vi "Sub05_MatlabFileBuilder.vi"(5 "Select line style":string(combo), 6 "Ball touch color":u32(colorbox), 7 "appended array":T2(array[cluster]), 8 "error in (no error)":errorcluster, 9 "Band touch color":u32(colorbox), 10 "CommandInfo":T1, 11 "Select sequence":string) -> (0 "error out":errorcluster, 3 "Script":string)   [LabVIEW 2019]
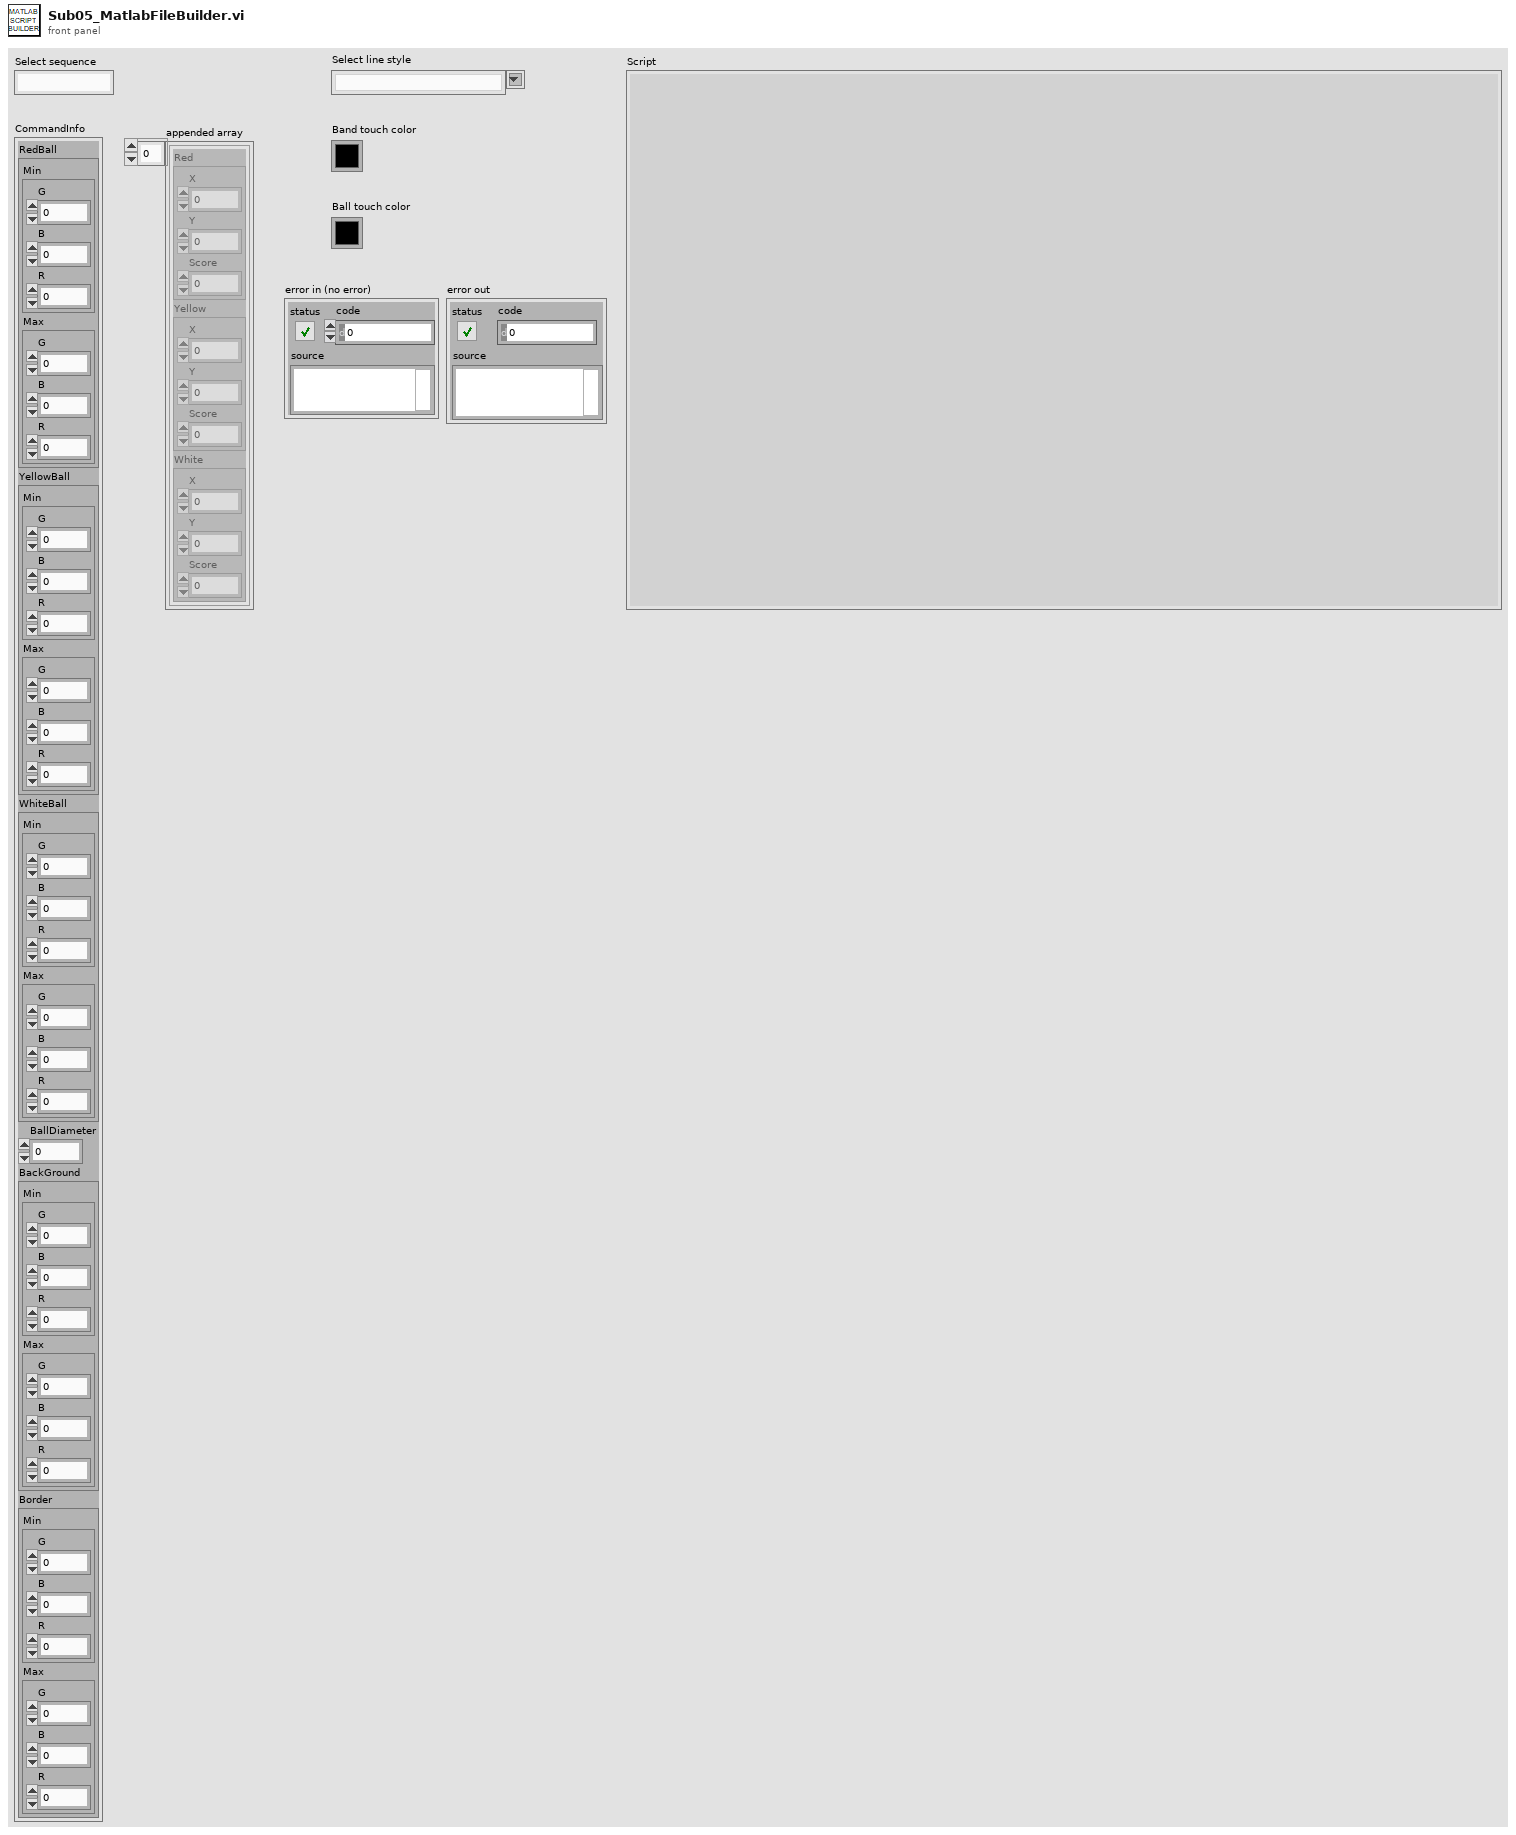
[diagram p1: front panel]
types:
  T1 = cluster{"RedBall":cluster{"Min":cluster{"G":u32, "B":u32, "R":u32}, "Max":cluster{"G":u32, "B":u32, "R":u32}}, "YellowBall":cluster{"Min":cluster{"G":u32, "B":u32, "R":u32}, "Max":cluster{"G":u32, "B":u32, "R":u32}}, "WhiteBall":cluster{"Min":cluster{"G":u32, "B":u32, "R":u32}, "Max":cluster{"G":u32, "B":u32, "R":u32}}, "BallDiameter":u32, "BackGround":cluster{"Min":cluster{"G":u32, "B":u32, "R":u32}, "Max":cluster{"G":u32, "B":u32, "R":u32}}, "Border":cluster{"Min":cluster{"G":u32, "B":u32, "R":u32}, "Max":cluster{"G":u32, "B":u32, "R":u32}}}
  T2 = cluster{"Red":cluster{"X":u32, "Y":u32, "Score":u32}, "Yellow":cluster{"X":u32, "Y":u32, "Score":u32}, "White":cluster{"X":u32, "Y":u32, "Score":u32}}[]
  T3 = cluster{"Min":cluster{"G":u32, "B":u32, "R":u32}, "Max":cluster{"G":u32, "B":u32, "R":u32}}
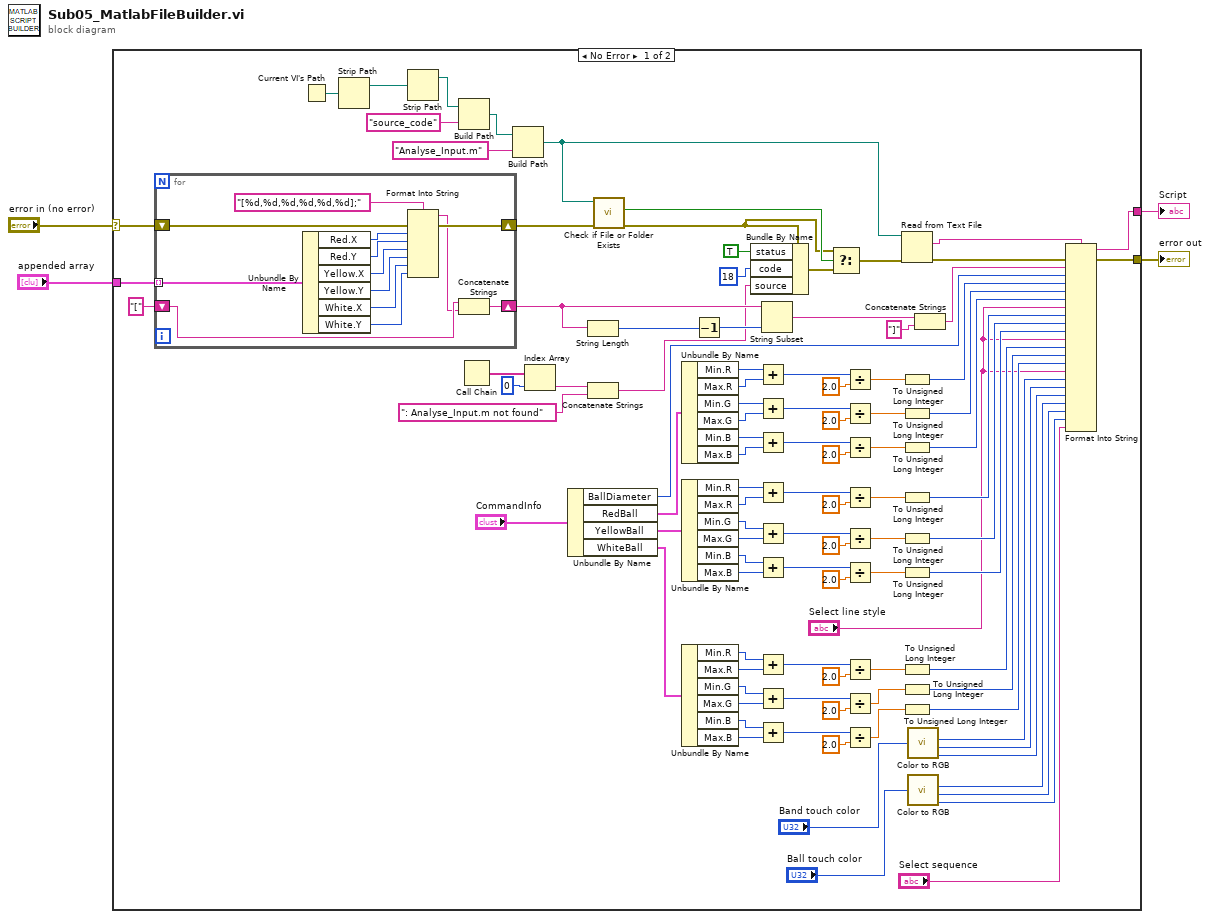
[diagram p0: block diagram]
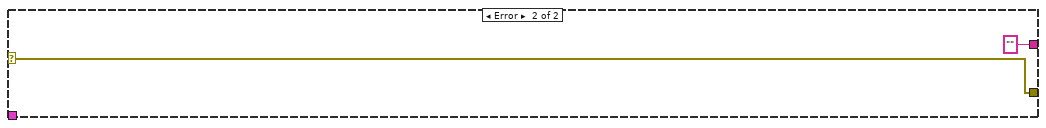
[diagram p2: hidden frame]
diagram:
  n1 = case shown="No Error" "error in (no error)" {
    selector: "error in (no error)" -> [w49 w119]
    tunnel: "appended array" -> [w98 _]
    tunnel: [w51 ""] -> w3
    tunnel: [w50 w119] -> w2
    frame No Error {
      n2 = for {
        tunnel: w98 -> [w118] mode=indexing
        shift-right: [w110] -> w102
        shift-left: "[" -> [w111]
        shift-right: [w108] -> w46
        shift-left: w49 -> [w109]
        n3 = Unbundle By Name(w118) -> ("Red.X"=w117:u32, "Red.Y"=w116:u32, "Yellow.X"=w115:u32, "Yellow.Y"=w114:u32, "White.X"=w113:u32, "White.Y"=w112:u32)
        n4 = Format Into String(format string="[%d,%d,%d,%d,%d,%d];" ("initial string"), error in=w109, w117, w116, w115, w114, w113, w112) -> (resulting string=w107:string, error out=w108:errorcluster)  [unwired: 1 in]
        n5 = Concatenate Strings(w111, w107) -> (w110:string)
      }
      n6 = Current VI's Path() -> (path=w52:path)
      n7 = Strip Path(path=w52) -> (stripped path=w35:path)  [unwired: 1 out]
      n8 = Strip Path(path=w35) -> (stripped path=w34:path)  [unwired: 1 out]
      n9 = Build Path(base path=w34, name or relative path="source_code") -> (appended path=w33:path)
      n10 = Call Chain() -> (call chain=w38:string[])
      n11 = Build Path(base path=w33, name or relative path="Analyse_Input.m") -> (appended path=w32:path)
      n12 = Index Array(array=w38, index=0) -> (element=w36:string)
      n13 = Unbundle By Name("CommandInfo") -> ("BallDiameter"=w55:u32, "RedBall"=w56:T3, "YellowBall"=w69:T3, "WhiteBall"=w82:T3)
      n14 = String Length(string=w102) -> (length=w104:i32)
      n15 = Concatenate Strings(w36, ": Analyse_Input.m not found" ("string")) -> (w40:string)
      n16 = call <vilib>:"Check if File or Folder Exists.vi"("error in (no error)"=w46, "path"=w32) -> ("error out"=w44:errorcluster, "file or folder exists?"=w47:bool)  [unwired: 7 in, 1 out]
      n17 = Unbundle By Name(w56) -> ("Min.R"=w66:u32, "Max.R"=w65:u32, "Min.G"=w62:u32, "Max.G"=w61:u32, "Min.B"=w58:u32, "Max.B"=w57:u32)
      n18 = Unbundle By Name(w69) -> ("Min.R"=w79:u32, "Max.R"=w78:u32, "Min.G"=w75:u32, "Max.G"=w74:u32, "Min.B"=w71:u32, "Max.B"=w70:u32)
      n19 = Unbundle By Name(w82) -> ("Min.R"=w92:u32, "Max.R"=w91:u32, "Min.G"=w88:u32, "Max.G"=w87:u32, "Min.B"=w84:u32, "Max.B"=w83:u32)
      n20 = Decrement(x=w104) -> (x-1=w103:i32)
      n21 = Bundle By Name(cluster=w44, "status"=TRUE, "code"=18, "source"=w40) -> (w39:errorcluster)
      n22 = Add(x=w66, y=w65) -> (x+y=w68:u32)
      n23 = Add(x=w62, y=w61) -> (x+y=w64:u32)
      n24 = Add(x=w58, y=w57) -> (x+y=w60:u32)
      n25 = Add(x=w79, y=w78) -> (x+y=w81:u32)
      n26 = Add(x=w75, y=w74) -> (x+y=w77:u32)
      n27 = Add(x=w71, y=w70) -> (x+y=w73:u32)
      n28 = Add(x=w92, y=w91) -> (x+y=w94:u32)
      n29 = Add(x=w88, y=w87) -> (x+y=w90:u32)
      n30 = Add(x=w84, y=w83) -> (x+y=w86:u32)
      n31 = String Subset(string=w102, length (rest)=w103) -> (substring=w101:string)  [unwired: 1 in]
      n32 = Select(t=w44, s=w47, f=w39) -> (s? t:f=w45:errorcluster)
      n33 = Divide(x=w68, y=2.0) -> (x/y=w30:dbl)
      n34 = Divide(x=w64, y=2.0) -> (x/y=w28:dbl)
      n35 = Divide(x=w60, y=2.0) -> (x/y=w26:dbl)
      n36 = Divide(x=w81, y=2.0) -> (x/y=w24:dbl)
      n37 = Divide(x=w77, y=2.0) -> (x/y=w22:dbl)
      n38 = Divide(x=w73, y=2.0) -> (x/y=w20:dbl)
      n39 = Divide(x=w94, y=2.0) -> (x/y=w18:dbl)
      n40 = Divide(x=w90, y=2.0) -> (x/y=w16:dbl)
      n41 = Divide(x=w86, y=2.0) -> (x/y=w14:dbl)
      n42 = Read from Text File(file (use dialog)=w32, error in=w45) -> (text=w54:string, error out=w53:errorcluster)  [unwired: 2 in, 2 out]
      n43 = To Unsigned Long Integer(number=w30) -> (unsigned 32bit integer=w29:u32)
      n44 = To Unsigned Long Integer(number=w28) -> (unsigned 32bit integer=w27:u32)
      n45 = To Unsigned Long Integer(number=w26) -> (unsigned 32bit integer=w25:u32)
      n46 = To Unsigned Long Integer(number=w24) -> (unsigned 32bit integer=w23:u32)
      n47 = To Unsigned Long Integer(number=w22) -> (unsigned 32bit integer=w21:u32)
      n48 = To Unsigned Long Integer(number=w20) -> (unsigned 32bit integer=w19:u32)
      n49 = To Unsigned Long Integer(number=w18) -> (unsigned 32bit integer=w17:u32)
      n50 = To Unsigned Long Integer(number=w16) -> (unsigned 32bit integer=w15:u32)
      n51 = To Unsigned Long Integer(number=w14) -> (unsigned 32bit integer=w13:u32)
      n52 = call <vilib>:"Color to RGB.vi"("Color"="Band touch color") -> ("R"=w12:u8, "G"=w11:u8, "B"=w10:u8)  [unwired: 1 out]
      n53 = call <vilib>:"Color to RGB.vi"("Color"="Ball touch color") -> ("R"=w9:u8, "G"=w8:u8, "B"=w7:u8)  [unwired: 1 out]
      n54 = Concatenate Strings(w101, "]" ("string")) -> (w99:string)
      n55 = Format Into String(format string=w54, error in=w53, w99, w55, w29, w27, w25, "Select line style", w23, w21, w19, "Select line style", w17, w15, w13, "Select line style", w12, w11, w10, w9, w8, w7, "Select sequence") -> (resulting string=w51:string, error out=w50:errorcluster)  [unwired: 1 in]
    }
    frame Error {
    }
  }
  "Script" <- w3
  "error out" <- w2
